vi "get_image_processor.vi"(8 "error in (no error)":errorcluster, 11 "GenericImageProcessorChangedCommand.lvclass in":refnum<class "GenericImageProcessorChangedCommand.lvclass">) -> (0 "error out":errorcluster, 2 "image processor":refnum<class "GenericImageProcessor.lvclass">, 3 "GenericImageProcessorChangedCommand.lvclass out":refnum<class "GenericImageProcessorChangedCommand.lvclass">)   [LabVIEW 2010, in "GenericImageProcessorChangedCommand.lvclass"]
uses:
  GenericImageProcessorChangedCommand.lvclass
  ImageProcessor/GenericImageProcessor/GenericImageProcessor/GenericImageProcessor.lvclass
  GenericImageProcessorChangedCommand.lvclass/GenericImageProcessorChangedCommand.ctl
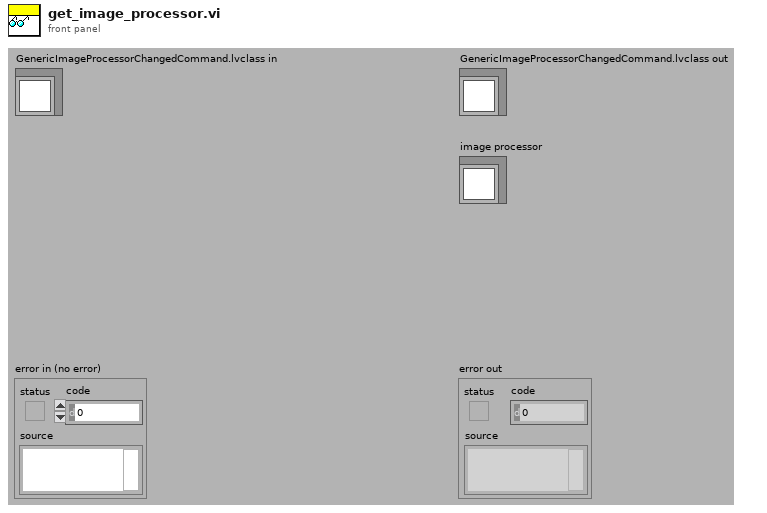
[diagram p1: front panel]
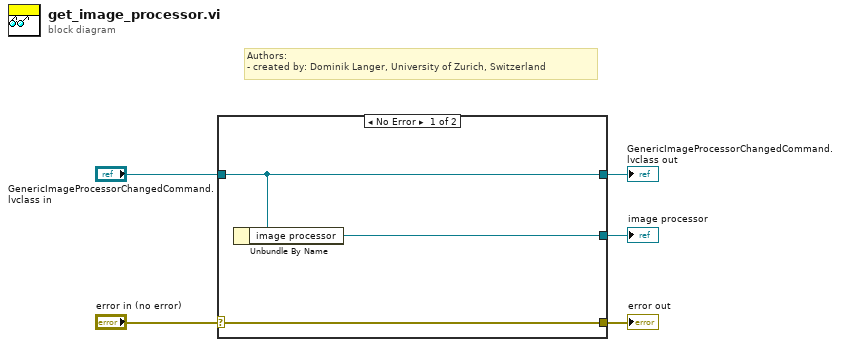
[diagram p0: block diagram]
diagram:
  # "Authors: \n- created by: Dominik Langer, University of Zurich, Switzerland"
  n1 = case shown="No Error" "error in (no error)" {
    selector: "error in (no error)" -> [w8 w9]
    tunnel: [w8 w9] -> w4
    tunnel: [w7 w10] -> w2
    tunnel: "GenericImageProcessorChangedCommand.lvclass in" -> [w7 w10]
    tunnel: [w6 _] -> w1
    frame No Error {
      n2 = Unbundle By Name(w7) -> ("image processor"=w6:refnum<class "GenericImageProcessor.lvclass">)
    }
    frame Error {
    }
  }
  "error out" <- w4
  "GenericImageProcessorChangedCommand.lvclass out" <- w2
  "image processor" <- w1
